vi "Connect_to_Arduino.vi"(8 "error in (no error)":errorcluster) -> (0 "error out":errorcluster, 2 "DISPOSITIVO CONECTADO":string, 3 "VISA Refnum out":refnum<visa-resource-name>)   [LabVIEW 2019, in "SHARED VI'S.lvlib"]
uses:
  SHARED VI'S.lvlib
  <vilib>/Utility/error.llb/Error Cluster From Error Code.vi
  <vilib>/Instr/_visa.llb/VISA Configure Serial Port (Instr).vi
  <vilib>/ErrorRing/Error Ring.xnode
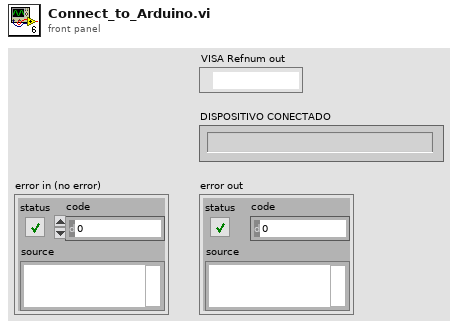
[diagram p1: front panel]
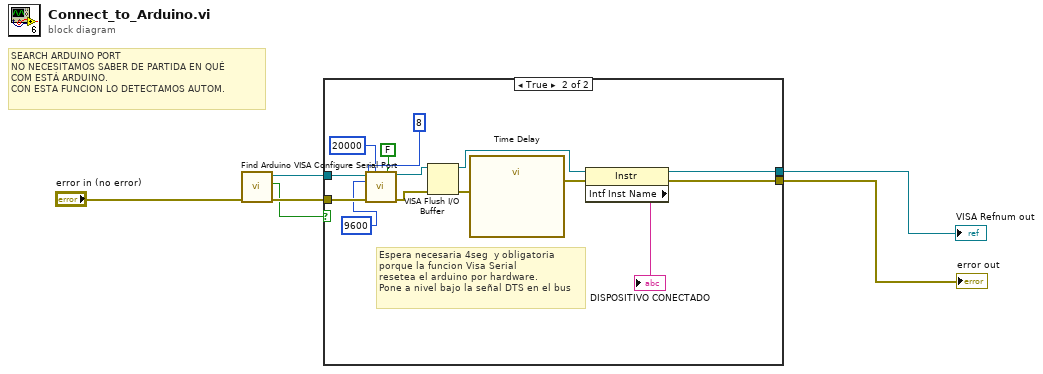
[diagram p0: block diagram]
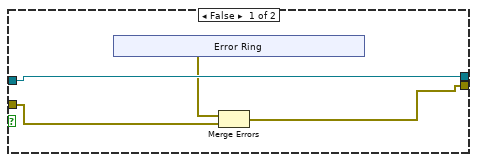
[diagram p2: hidden frame]
diagram:
  # "SEARCH ARDUINO PORT\nNO NECESITAMOS SABER DE PARTIDA EN QUÉ\nCOM ESTÁ ARDUINO. \nCON ESTA FUNCION LO DETECTAMOS AUTOM."
  n1 = call "Find Arduino.vi"("error in (no error)"="error in (no error)") -> ("error out"=w2:errorcluster, "Arduino Found?"=w1:bool, "VISA resource name"=w3:refnum<visa-resource-name>)  [unwired: 8 in]
  n2 = case shown="True" w1 {
    tunnel: [w7 w29] -> w6
    tunnel: [w10 w27] -> w5
    tunnel: w3 -> [w10 w24]
    tunnel: w2 -> [w8 w23]
    frame False {
      n3 = xnode "Error Ring"() -> ("error out"=w9:errorcluster)
      n4 = Merge Errors(w9, w8) -> (w7:errorcluster)
    }
    frame True {
      # "Espera necesaria 4seg  y obligatoria\nporque la funcion Visa Serial\nresetea el arduino por hardware.\nPone a nivel bajo la señal DTS en el bus"
      n5 = call-poly "VISA Configure Serial Port"("VISA resource name"=w24, "timeout (10sec)"=u32 20000, "Enable Termination\nChar (T)"=FALSE ("Enable Termination\nChar (T)"), "baud rate (9600)"=u32 9600, "data bits (8)"=u16 8, "error in (no error)"=w23) -> ("VISA resource name out"=w20:refnum<visa-resource-name>, "error out"=w19:errorcluster)  [unwired: 8 in]
      n6 = VISA Flush I/O Buffer(VISA resource name=w20, error in (no error)=w19) -> (VISA resource name out=w17:refnum<visa-resource-name>, error out=w18:errorcluster)  [unwired: 1 in]
      n7 = call "Time Delay"("error in (no error)"=w18) -> ("error out"=w28:errorcluster)  [unwired: 10 in]
      n8 = property class="Instr"(reference=w17, error in=w28) -> (reference out=w27:refnum<visa-resource-name>, error out=w29:errorcluster, "Intf Inst Name"=→"DISPOSITIVO CONECTADO":string)
    }
  }
  "error out" <- w6
  "VISA Refnum out" <- w5
